vi "Generate Trace.vi"(11 "String":string) -> ()   [LabVIEW 2020, in "Actor Framework.lvlib"]
uses:
  ActorFramework/Actor Framework.lvlib
  ActorFramework/tracing/AF Trace Format/AF Trace Format.lvclass
  <resource>/dialog/lvconfig.llb/LV Config Read String.vi
  <vilib>/Utility/SystemLogging/NI_SystemLogging.lvlib
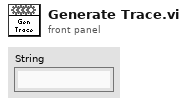
[diagram p1: front panel]
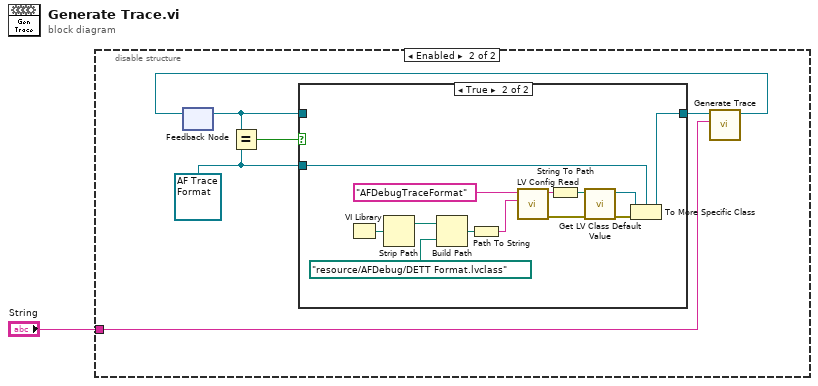
[diagram p0: block diagram]
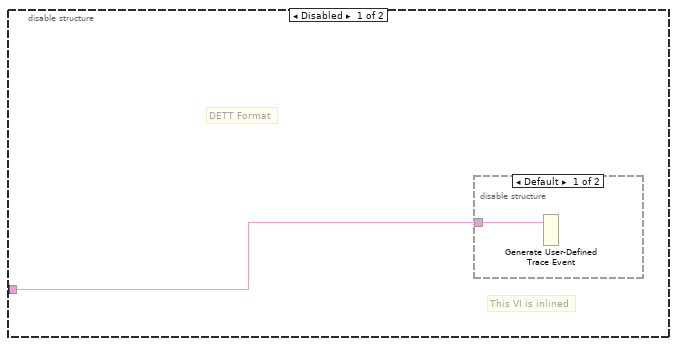
[diagram p2: hidden frame]
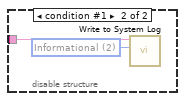
[diagram p3: hidden frame]
diagram:
  n1 = disable-structure shown="Enabled" {
    disable-tunnel: "String" -> [w2 w6]
    frame Disabled {
      # "DETT Format"
      # "This VI is inlined"
      n2 = disable-structure shown="Default" {
        disable-tunnel: w2 -> [w3 w5]
        frame condition #0 (active) {
          n3 = Generate User-Defined Trace Event(2:w3) -> ()  [unwired: 1 in]
        }
        frame condition #1 {
          w4 = 2 items=["Error", "Warning", "Informational"] ("severity")
          n4 = call <vilib>:"Write to System Log.vi"("severity"=w4, "message"=w5) -> ()  [unwired: 9 in, 1 out]
        }
      }
    }
    frame Enabled {
      w8 = refnum<class "AF Trace Format.lvclass"> refnum ("Actor Framework:AF Trace Format.lvclass")
      n5 = feedback #1() -> (w11:refnum<class "AF Trace Format.lvclass">)  [unwired: 1 in]
      n6 = Equal?(x=w11, y=w8) -> (x = y?=w10:bool)
      n7 = case shown="True" w10 {
        tunnel: w11 -> [w12 _]
        tunnel: [w12 w13] -> w9
        tunnel: w8 -> [_ w14]
        frame False {
        }
        frame True {
          n8 = VI Library() -> (path=w24:path)
          n9 = Strip Path(path=w24) -> (stripped path=w23:path)  [unwired: 1 out]
          n10 = Build Path(base path=w23, name or relative path=path "resource/AFDebug/DETT Format.lvclass") -> (appended path=w21:path)
          n11 = Path To String(path=w21) -> (string=w20:string)
          n12 = call-poly <resource>:"LV Config Read.vi"("default value"=w20, "key"="AFDebugTraceFormat") -> ("error out"=w19:errorcluster, "value"=w17:string)  [unwired: 3 in, 1 out]
          n13 = String To Path(string=w17) -> (path=w18:path)
          n14 = call <vilib>:"Get LV Class Default Value.vi"("error in (no error)"=w19, "class path"=w18) -> ("error out"=w16:errorcluster, "object"=w15:refnum<class>)  [unwired: 8 in]
          n15 = To More Specific Class(target class=w14, reference=w15, error in=w16) -> (specific class reference=w13:refnum<class "AF Trace Format.lvclass">)  [unwired: 1 out]
        }
      }
      n16 = call-dynamic "Generate Trace.vi"("Trace String"=w6, "AF Trace Format in"=w9) -> ("AF Trace Format out"=w7:refnum<class "AF Trace Format.lvclass">)  [unwired: 9 in]
      n17 = feedback-in #1(w7) -> ()
    }
  }
